vi "R5SBRControl_Status.vi"(7 "LabVIEW Web Service Request":refnum<class "Web Request.lvclass">) -> (0 "error out":errorcluster)   [LabVIEW 2016]
uses:
  <vilib>/wsapi/Web Request.lvclass
  R5Controls/R5SBR_Status.ctl
  R5Controls/R5SBR_SetParams.ctl
panel:
  # "Use the Web Service Request input terminal to call the VIs on the Web Services palette. Do not remove it from the connector pane unless you don't need access to the palette."
  # "Each additional control wired to the connector pane will be available as an input in the URL. To include an indicator in terminal-mode output (the default setting), it must also be wired to the connector pane."
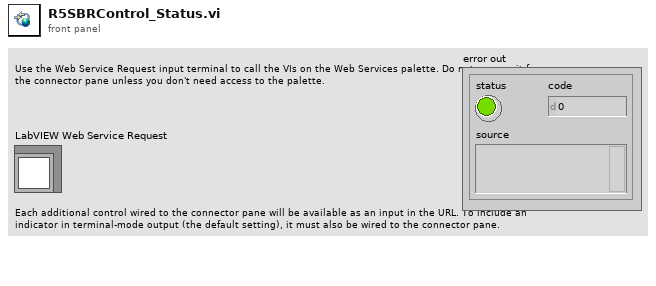
[diagram p1: front panel]
types:
  T1 = typedef "R5SBR_Status.ctl" = cluster{"SBR_Switch":bool, "SBR_Outputs":cluster{"Cycle Time Elapsed, min":dbl, "Phase Time Elapsed, min":dbl, "Timestamp":string, "Status":string}, "SBR_Manual":cluster{"Influent Pump":bool, "Effluent Pump":bool}, "R5SBR_SetParams":T2}
  T2 = typedef "R5SBR_SetParams.ctl" = cluster{"Phase":string, "Time, min":dbl, "SBR_Manual":cluster{"Influent Pump":bool, "Effluent Pump":bool}}[]
  T3 = cluster{"Phase":string, "Time, min":dbl, "SBR_Manual":cluster{"Influent Pump":bool, "Effluent Pump":bool}}[]
  T4 = cluster{"Influent Pump":bool, "Effluent Pump":bool}
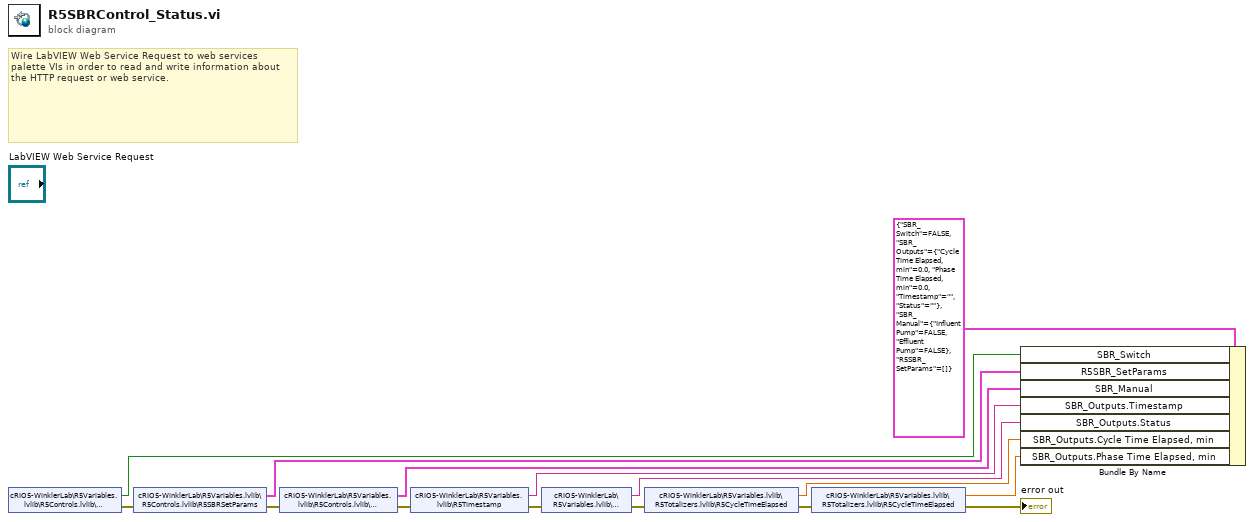
[diagram p0: block diagram]
diagram:
  # "Wire LabVIEW Web Service Request to web services palette VIs in order to read and write information about the HTTP request or web service."
  n1 = shared-variable "cRIO5-WinklerLab\\R5Variables.lvlib\\R5Controls.lvlib\\R5SBRSwitch"() -> (w7:bool, error out=w14:errorcluster)  [unwired: 1 in]
  n2 = shared-variable "cRIO5-WinklerLab\\R5Variables.lvlib\\R5Controls.lvlib\\R5SBRSetParams"(error in=w14) -> (w6:T3, error out=w13:errorcluster)
  n3 = shared-variable "cRIO5-WinklerLab\\R5Variables.lvlib\\R5Controls.lvlib\\R5SBRManual"(error in=w13) -> (w5:T4, error out=w12:errorcluster)
  n4 = shared-variable "cRIO5-WinklerLab\\R5Variables.lvlib\\R5Timestamp"(error in=w12) -> (w4:string, error out=w11:errorcluster)
  n5 = shared-variable "cRIO5-WinklerLab\\R5Variables.lvlib\\R5Status"(error in=w11) -> (w3:string, error out=w10:errorcluster)
  n6 = shared-variable "cRIO5-WinklerLab\\R5Variables.lvlib\\R5Totalizers.lvlib\\R5CycleTimeElapsed"(error in=w10) -> (w2:dbl, error out=w9:errorcluster)
  n7 = shared-variable "cRIO5-WinklerLab\\R5Variables.lvlib\\R5Totalizers.lvlib\\R5CycleTimeElapsed"(error in=w9) -> (w1:dbl, error out=→"error out":errorcluster)
  n8 = Bundle By Name(cluster=T1 {"SBR_Switch"=FALSE, "SBR_Outputs"={"Cycle Time Elapsed, min"=0.0, "Phase Time Elapsed, min"=0.0, "Timestamp"="", "Status"=""}, "SBR_Manual"={"Influent Pump"=FALSE, "Effluent Pump"=FALSE}, "R5SBR_SetParams"=[]} ("SBRData"), "SBR_Switch"=w7, "R5SBR_SetParams"=w6, "SBR_Manual"=w5, "SBR_Outputs.Timestamp"=w4, "SBR_Outputs.Status"=w3, "SBR_Outputs.Cycle Time Elapsed, min"=w2, "SBR_Outputs.Phase Time Elapsed, min"=w1) -> ()  [unwired: 1 out]
